vi "Configure  Results Display.vi"(8 "error IO":errorcluster, 10 "Results Display":enum16{"Last", "ALL", "P/F"}(ring), 11 "VISA resource name":refnum<visa-resource-name>) -> (0 "error Out":errorcluster, 3 "VISA resource Out":refnum<visa-resource-name>)   [LabVIEW 2016, in "eec EST 300.lvlib"]
doc: "SR <status>\nSets the Results Display setting. This allows you to set the results display after a test sequence has been run. There are 3 options:\n\n0=Last: a Results summary screen will be displayed at the end of the test or sequence of connected steps displaying the results of all of the steps.\n1=AllL: the results of the last step performed will be displayed on the Perform Tests screen.\n2=P/F: a Pass or Fail screen will be displayed at the end of the test."
uses:
  <instrlib>/eec EST 300/eec EST 300.lvlib
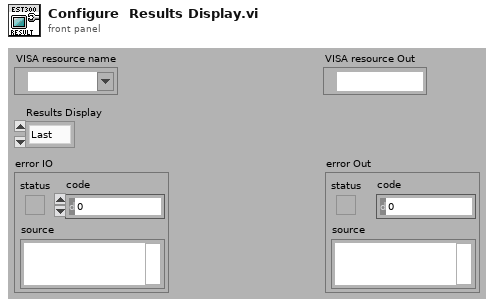
[diagram p1: front panel]
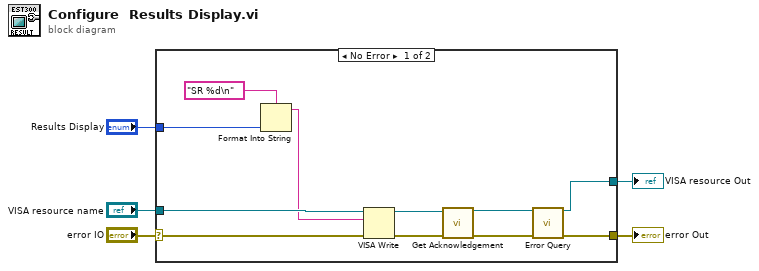
[diagram p0: block diagram]
diagram:
  n1 = case shown="No Error" "error IO" {
    selector: "error IO" -> [w16 w18]
    tunnel: [w13 w18] -> w2
    tunnel: [w14 w17] -> w3
    tunnel: "VISA resource name" -> [w15 w17]
    tunnel: "Results Display" -> [w7 _]
    frame No Error {
      n2 = Format Into String(format string="SR %d\n" ("Command to Send (empty)"), w7) -> (resulting string=w6:string)  [unwired: 2 in, 1 out]
      n3 = VISA Write(VISA resource name=w15, write buffer=w6, error in (no error)=w16) -> (VISA resource name out=w9:refnum<visa-resource-name>, error out=w10:errorcluster)  [unwired: 1 out]
      n4 = call <instrlib>:"Get Acknowledgement.vi"("VISA resource name"=w9, "error in (no error)"=w10) -> ("VISA resource name out"=w12:refnum<visa-resource-name>, "error out"=w11:errorcluster)  [unwired: 12 in]
      n5 = call <instrlib>:"Error Query.vi"("VISA resource name"=w12, "error in (no error)"=w11) -> ("VISA resource name out"=w14:refnum<visa-resource-name>, "error out"=w13:errorcluster)  [unwired: 10 in, 2 out]
    }
    frame Error {
    }
  }
  "VISA resource Out" <- w3
  "error Out" <- w2
